vi "MatchConfig.vi"(8 "error in (no error)":errorcluster, 10 "Selected Channels":T3=[0], 11 "9213 in":refnum<class "9213.lvclass">) -> (0 "error out":errorcluster, 1 "All same DegreeRange?":bool, 2 "DegreeRange value":T1 items=["Raw Volts", "Degrees Kelvin", "Degrees Celsius", "Degrees Fahrenheit", "Degrees Rankine"], 3 "9213 out":refnum<class "9213.lvclass">, 4 "TCoupleType value":T2 items=["J", "K", "T", "E", "R", "S", "N", "B"], 6 "All same TCoupleType?":bool)   [LabVIEW 2011, in "Modules.lvlib" / "9213.lvclass"]
uses:
  9213.lvclass
  Channels Listbox.ctl
  Thermocouple Type.ctl
  Measurement Units.ctl
  9213.lvclass/9213.ctl
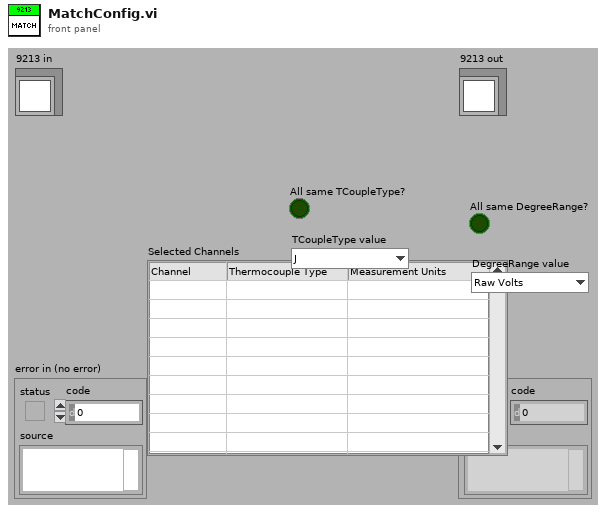
[diagram p1: front panel]
types:
  T1 = typedef "Modules.lvlib/9213.lvclass/Measurement Units.ctl" = u8
  T2 = typedef "Modules.lvlib/9213.lvclass/Thermocouple Type.ctl" = u8
  T3 = typedef "Modules.lvlib/9213.lvclass/Channels Listbox.ctl" = i32[]
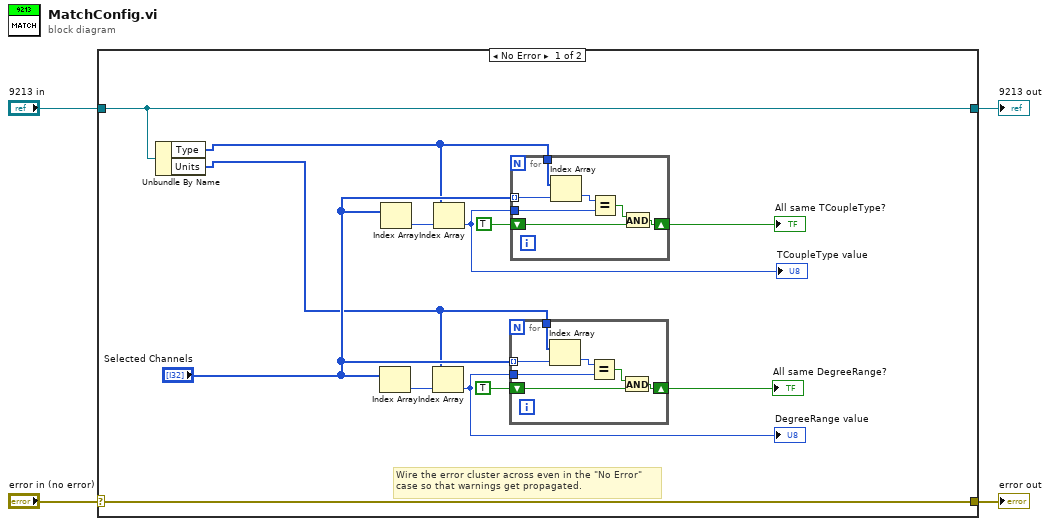
[diagram p0: block diagram]
diagram:
  n1 = case shown="No Error" "error in (no error)" {
    selector: "error in (no error)" -> [w17 w33]
    tunnel: [w17 w33] -> w3
    tunnel: [w7 w32] -> w1
    tunnel: "9213 in" -> [w7 w32]
    frame No Error {
      # "Wire the error cluster across even in the \"No Error\"\ncase so that warnings get propagated."
      n2 = Unbundle By Name(w7) -> ("Type"=w5:T2[], "Units"=w6:T1[])
      n3 = Index Array(array="Selected Channels") -> (element=w9:i32)  [unwired: 1 in]
      n4 = Index Array(array="Selected Channels") -> (element=w10:i32)  [unwired: 1 in]
      n5 = Index Array(array=w6, index=w9) -> (element=w13:T1)
      "DegreeRange value" <- w13
      n6 = Index Array(array=w5, index=w10) -> (element=w16:T2)
      "TCoupleType value" <- w16
      n7 = for {
        tunnel: "Selected Channels" -> [w23] mode=indexing
        tunnel: w6 -> [w24]
        tunnel: w13 -> [w21]
        shift-right: [w19] -> w12
        shift-left: TRUE -> [w18]
        n8 = Index Array(array=w24, index=w23) -> (element=w22:T1)
        n9 = Equal?(x=w22, y=w21) -> (x = y?=w20:bool)
        n10 = And(x=w20, y=w18) -> (x .and. y?=w19:bool)
      }
      "All same DegreeRange?" <- w12
      n11 = for {
        tunnel: "Selected Channels" -> [w30] mode=indexing
        tunnel: w5 -> [w31]
        tunnel: w16 -> [w28]
        shift-right: [w26] -> w15
        shift-left: TRUE -> [w25]
        n12 = Index Array(array=w31, index=w30) -> (element=w29:T2)
        n13 = Equal?(x=w29, y=w28) -> (x = y?=w27:bool)
        n14 = And(x=w27, y=w25) -> (x .and. y?=w26:bool)
      }
      "All same TCoupleType?" <- w15
    }
    frame Error {
    }
  }
  "error out" <- w3
  "9213 out" <- w1
